vi "Cut Selection.vi"   [LabVIEW 2019]
doc: "Demonstrates the Cut Selection method in VI Scripting, which places the selected portion of a VI on the system clipboard. It has the same effect as choosing Edit > Cut from the user interface."
panel:
  # "Overview: Demonstrates the Cut Selection method in VI Scripting, which places the selected portion of a VI on the system clipboard.\nInstructions:\n1. Open the block diagram of Test - Selection List Target.vi.\n2. Select one or more objects.\n3. Run this VI. The selected objects will be cut to the system clipboard.\n4. Open a new VI block diagram.\n5. Select Edit > Paste from the menu bar. The items you originally selected (which were programmatically cut to the clipboard) will be pasted onto the new VI block diagram."
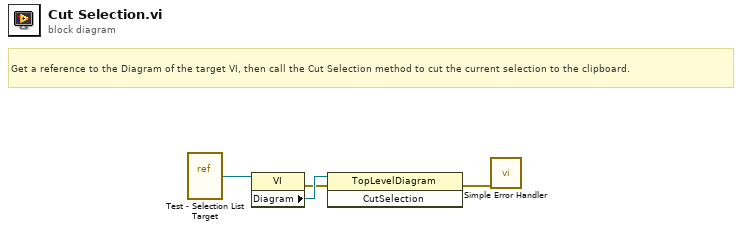
[diagram p0: block diagram]
diagram:
  # "Get a reference to the Diagram of the target VI, then call the Cut Selection method to cut the current selection to the clipboard."
  n1 = vi-ref "Test - Selection List Target.vi"() -> (w4:refnum<vi>)
  n2 = property class="VI"(reference=w4) -> (error out=w2:errorcluster, "Diagram"=w3:refnum<vi>)  [unwired: 1 in, 1 out]
  n3 = invoke class="TopLevelDiagram" method="CutSelection"(reference=w3, error in=w2) -> (error out=w1:errorcluster)  [unwired: 1 in, 2 out]
  n4 = call <vilib>:"Simple Error Handler.vi"("error in (no error)"=w1) -> ()  [unwired: 4 in, 5 out]
